vi "Search Consumer Information Array.vi"(8 "error in (no error)":errorcluster, 10 "Consumer in":string, 11 "Consumer Information Array in":T1[](array[typedef])) -> (0 "error out":errorcluster, 3 "Consumer Information out":T1)   [LabVIEW 2027, in "Messaging.lvlib" / "Abstract Producer.lvclass"]
uses:
  Abstract Producer.lvclass
  Consumer Information.ctl
  Message Queue/Abstract Message Queue/Abstract Message Queue.lvclass
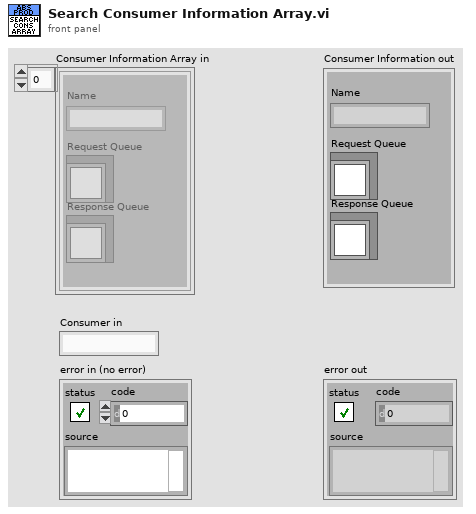
[diagram p1: front panel]
types:
  T1 = typedef "Messaging.lvlib/Abstract Producer.lvclass/Consumer Information.ctl" = cluster{"Name":string, "Request Queue":refnum<class "Abstract Message Queue.lvclass">, "Response Queue":refnum<class "Abstract Message Queue.lvclass">}
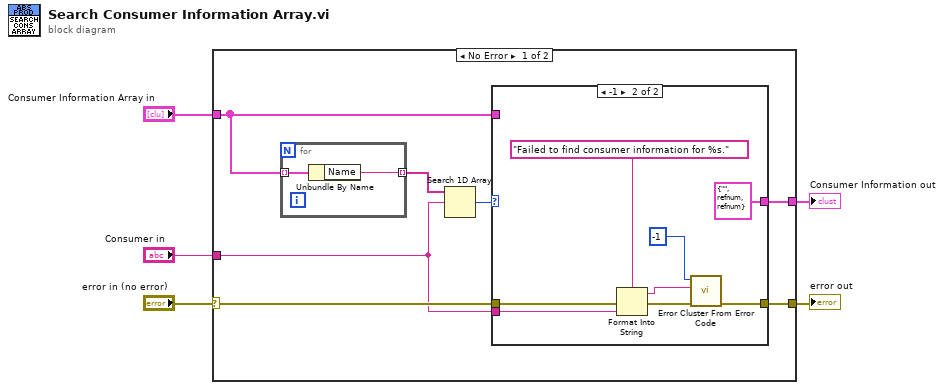
[diagram p0: block diagram]
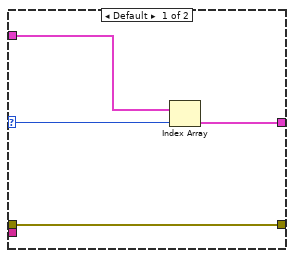
[diagram p2: hidden frame]
diagram:
  n1 = case shown="No Error" "error in (no error)" {
    selector: "error in (no error)" -> [w7 w27]
    tunnel: "Consumer in" -> [w6 _]
    tunnel: "Consumer Information Array in" -> [w11 _]
    tunnel: [w9 _] -> w3
    tunnel: [w8 w27] -> w2
    frame No Error {
      n2 = for {
        tunnel: w11 -> [w26] mode=indexing
        tunnel: [w25] -> w12 mode=indexing
        n3 = Unbundle By Name(w26) -> ("Name"=w25:string)
      }
      n4 = Search 1D Array(1D array=w12, element=w6) -> (index of element=w10:i32)  [unwired: 1 in]
      n5 = case shown="-1" w10 {
        selector: w10 -> [w15 _]
        tunnel: w11 -> [w16 _]
        tunnel: [w14 T1 {"Name"="", "Request Queue"=refnum, "Response Queue"=refnum} ("Consumer Information")] -> w9
        tunnel: w7 -> [w13 w21]
        tunnel: [w13 w23] -> w8
        tunnel: w6 -> [_ w19]
        frame Default {
          n6 = Index Array(array=w16, index=w15) -> (element=w14:T1)
        }
        frame -1 {
          n7 = Format Into String(format string="Failed to find consumer information for %s.", error in=w21, w19) -> (resulting string=w18:string, error out=w20:errorcluster)  [unwired: 1 in]
          n8 = call <vilib>:"Error Cluster From Error Code.vi"("error in (no error)"=w20, "error message (\"\")"=w18, "error code (0)"=-1) -> ("error out"=w23:errorcluster)  [unwired: 6 in]
        }
      }
    }
    frame Error {
    }
  }
  "Consumer Information out" <- w3
  "error out" <- w2
